vi "Write DVR_PLC Fault.vi"(8 "error in (no error)":errorcluster, 10 "DVR_PLC Fault":refnum<data-value>, 11 "OPC UA in":refnum<class "OPC UA.lvclass">) -> (0 "error out":errorcluster, 3 "OPC UA out":refnum<class "OPC UA.lvclass">)   [LabVIEW 2021, in "OPC UA.lvlib" / "OPC UA.lvclass"]
uses:
  OPC UA.lvclass
  OPC UA.lvclass/OPC UA.ctl
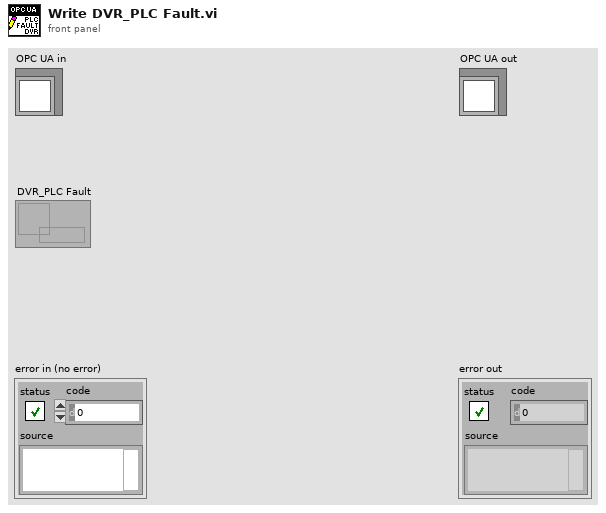
[diagram p1: front panel]
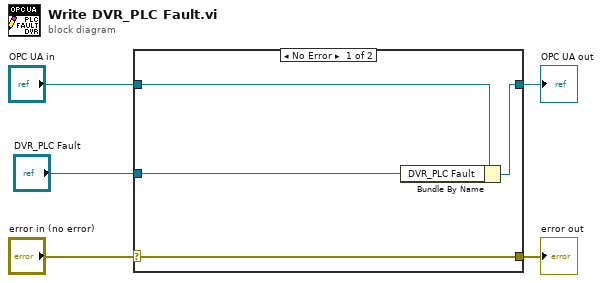
[diagram p0: block diagram]
diagram:
  n1 = case shown="No Error" "error in (no error)" {
    selector: "error in (no error)" -> [w9 w10]
    tunnel: [w9 w10] -> w4
    tunnel: [w7 w11] -> w2
    tunnel: "OPC UA in" -> [w8 w11]
    tunnel: "DVR_PLC Fault" -> [w6 _]
    frame No Error {
      n2 = Bundle By Name(cluster=w8, "DVR_PLC Fault"=w6) -> (w7:refnum<class "OPC UA.lvclass">)
    }
    frame Error {
    }
  }
  "error out" <- w4
  "OPC UA out" <- w2
